vi "ShouldWeAdjustAngle.vi"(10 "DesiredHeading (0-360)":dbl, 11 "RobotHeading (0-360)":dbl) -> (3 "ShouldWeAdjustAngle?":bool)   [LabVIEW 2013]
doc: "Determines whether the robot heading should be adjusted. Returns true if the difference between the robot heading and the desired heading are greater than a given difference cutoff.\n\nBonnie Ishiguro\nSpring 2014"
uses:
  Utilities/Math/Angles/Angle/Angle.lvclass
panel:
  in  "DifferenceCutoff":i32=10
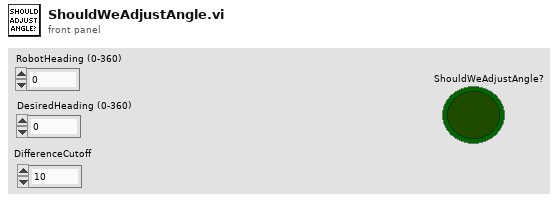
[diagram p1: front panel]
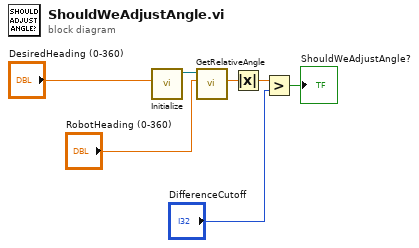
[diagram p0: block diagram]
diagram:
  n1 = call "Initialize.vi"("Input Angle (Deg.)"="DesiredHeading (0-360)") -> ("Angle out"=w7:refnum<class "Angle.lvclass">)  [unwired: 9 in, 1 out]
  n2 = call "GetRelativeAngle.vi"("Boat Heading (Deg.)"="RobotHeading (0-360)", "Angle in"=w7) -> ("Relative Angle FROM P2 TO P1 (deg)"=w2:dbl)  [unwired: 6 in, 3 out]
  n3 = Absolute Value(x=w2) -> (abs(x)=w1:dbl)
  n4 = Greater?(x=w1, y="DifferenceCutoff") -> (0:→"ShouldWeAdjustAngle?":bool)
